vi "Factorial.vi"(4 "N":i32) -> (1 "N!":dbl)   [LabVIEW 2011]
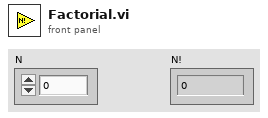
[diagram p1: front panel]
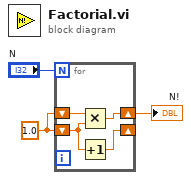
[diagram p0: block diagram]
diagram:
  w2 = 1.0
  n1 = for {
    N: "N" -> [_]
    shift-right: [w6] -> w1
    shift-left: w2 -> [w7]
    shift-right: [w5] -> _
    shift-left: w2 -> [w4]
    n2 = Multiply(x=w7, y=w4) -> (x*y=w6:dbl)
    n3 = Increment(x=w4) -> (x+1=w5:dbl)
  }
  "N!" <- w1
